vi "Get Child Text.vi"(0 "Item File Path":path, 5 "Node Type":string, 7 "Node URL":string) -> (4 "Child Text":string[](array[string]))   [LabVIEW 2016]
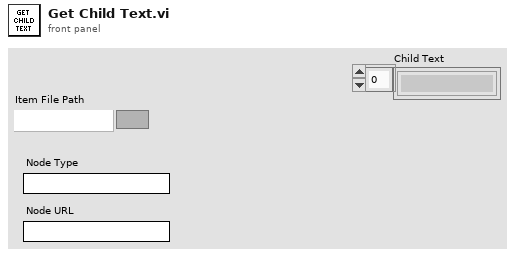
[diagram p1: front panel]
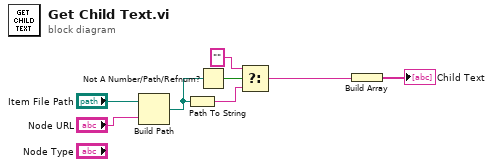
[diagram p0: block diagram]
diagram:
  n1 = Build Path(base path="Item File Path", name or relative path="Node URL") -> (appended path=w4:path)
  n2 = Path To String(path=w4) -> (string=w6:string)
  n3 = Not A Number/Path/Refnum?(number/path/refnum=w4) -> (NaN/Path/Refnum?=w7:bool)
  n4 = Select(t="", s=w7, f=w6) -> (s? t:f=w1:string)
  n5 = Build Array(w1) -> (→"Child Text":string[])
